vi "Update VeriStand Channel Values.vi"(8 "SignalIds Out":i32[](array[numeric]), 9 "SignalIds In":i32[](array[numeric]), 10 "Outport Channel refs":T1[](array[typedef]) format="%.0x", 11 "Inport Channel refs":T1[](array[typedef]) format="%.0x") -> ()   [LabVIEW 2026, in "Runtime Configuration Support Example Engine.lvlib"]
uses:
  <vilib>/NI VeriStand/Custom Device API/Custom Device Item Ref.ctl
  HW Operations.ctl
  <vilib>/NI VeriStand/Custom Device API/Global Data Refs.vi
  Runtime Configuration Support Example Engine.lvlib
  <vilib>/NI VeriStand/Custom Device API/Custom Device API.lvlib
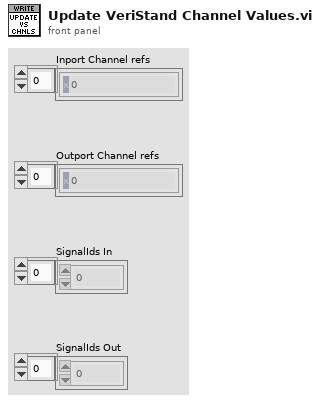
[diagram p1: front panel]
types:
  T1 = typedef "Custom Device API.lvlib/Custom Device Item Ref.ctl" = u64
  T2 = typedef "HW Operations.ctl" = enum16{"Initialize", "Set In Val", "Get In Val", "Set Block", "Set Out Val", "Get Out Val", "Get In Array", "Get Out Array"}
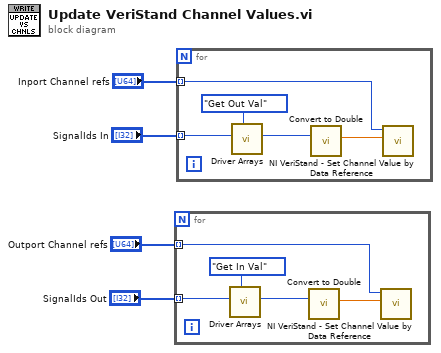
[diagram p0: block diagram]
diagram:
  n1 = for {
    tunnel: "SignalIds Out" -> [w8] mode=indexing
    tunnel: "Outport Channel refs" -> [w5] mode=indexing
    n2 = call "Driver Arrays.vi"("Index"=w8, "Curr Operation"=HW_Operations."Get In Val") -> ("Value"=w7:i32)  [unwired: 6 in, 3 out]
    n3 = call "Convert to Double.vi"("In"=w7) -> ("Out"=w6:dbl)  [unwired: 9 in, 1 out]
    n4 = call <vilib>:"NI VeriStand - Set Channel Value by Data Reference.vi"("Value"=w6, "Data Reference in"=w5) -> ()  [unwired: 9 in, 1 out]
  }
  n5 = for {
    tunnel: "SignalIds In" -> [w13] mode=indexing
    tunnel: "Inport Channel refs" -> [w10] mode=indexing
    n6 = call "Driver Arrays.vi"("Index"=w13, "Curr Operation"=HW_Operations."Get Out Val") -> ("Value"=w12:i32)  [unwired: 6 in, 3 out]
    n7 = call "Convert to Double.vi"("In"=w12) -> ("Out"=w11:dbl)  [unwired: 9 in, 1 out]
    n8 = call <vilib>:"NI VeriStand - Set Channel Value by Data Reference.vi"("Value"=w11, "Data Reference in"=w10) -> ()  [unwired: 9 in, 1 out]
  }
